vi "SynapseAPI-Set Parameter Value (bool).vi"(0 "URL":string="http://localhost:24414", 5 "Gizmo":string, 7 "Parameter":string, 9 "Value":bool, 11 "error in (no error)":errorcluster) -> (15 "error out":errorcluster)   [LabVIEW 2020]
uses:
  <vilib>/httpClient/PUTBuffer.vi
  <vilib>/httpClient/LabVIEWHTTPClient.lvlib
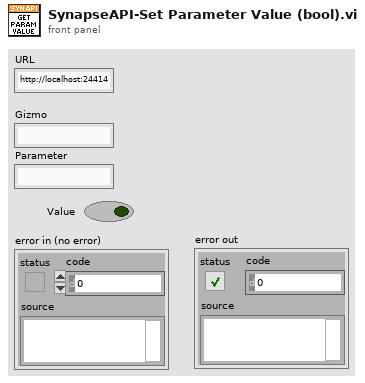
[diagram p1: front panel]
types:
  T1 = typedef "LabVIEWHTTPClient.lvlib/ClientHandle.ctl" = refnum<k1>
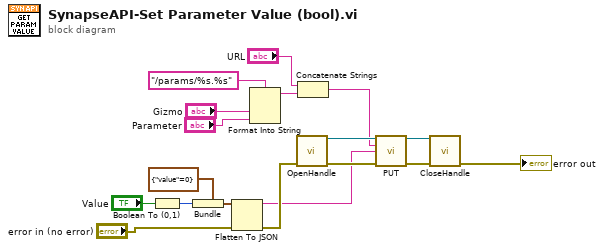
[diagram p0: block diagram]
diagram:
  n1 = Boolean To (0,1)(Boolean="Value") -> (0, 1=w5:i16)
  n2 = Bundle(cluster=cluster{"value":i32} {"value"=0} ("Cluster"), "value"=w5) -> (w4:cluster{"value":i32})
  n3 = Flatten To JSON(anything=w4, error in (no error)="error in (no error)") -> (JSON string=w1:string, 11:w2:errorcluster)  [unwired: 1 in]
  n4 = Format Into String(format string="/params/%s.%s", "Gizmo", "Parameter") -> (resulting string=w12:string)  [unwired: 2 in, 1 out]
  n5 = call <vilib>:"OpenHandle.vi"("error in (no error)"=w2) -> ("client handle out"=w16:T1, "error out"=w15:errorcluster)  [unwired: 13 in]
  n6 = Concatenate Strings("URL", w12) -> (w14:string)
  n7 = call-poly <vilib>:"PUT.vi"("client handle"=w16, "url"=w14, "buffer"=w1, "error in (no error)"=w15) -> ("client handle out"=w17:T1, "error out"=w18:errorcluster)  [unwired: 8 in, 2 out]
  n8 = call <vilib>:"CloseHandle.vi"("client handle"=w17, "error in (no error)"=w18) -> ("error out"=→"error out":errorcluster)  [unwired: 13 in]
